vi "KE622x -- Get Trace Buf Elements.vi"(0 "Resource In":refnum<visa-resource-name>, 1 "Check For SCPI Errors? (T)":bool=TRUE, 11 "error in (no error)":errorcluster) -> (4 "Resource Out (dupl)":refnum<visa-resource-name>, 8 "Meas Elements To Return":T1={"Timstamp?"=TRUE, "Reading Num?"=FALSE, "Source Value?"=FALSE, "Compliance?"=TRUE, "Average Voltage?"=FALSE}, 15 "error out":errorcluster)   [LabVIEW 2019, in "Keithley 622x.lvlib"]
uses:
  Keithley 622x.lvlib
  Format/Typedefs/KE622x -- Optional Meas Elements.ctl
panel:
  # "*** NOTE:  \"Average Voltage\"\nis only available for Differential\nConductance measurements."
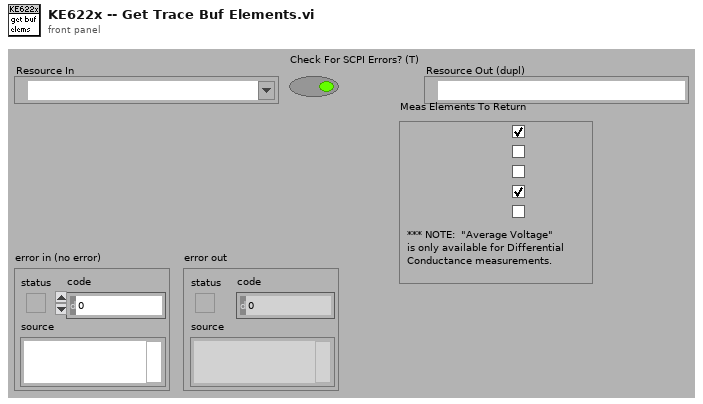
[diagram p1: front panel]
types:
  T1 = typedef "Keithley 622x.lvlib/KE622x -- Optional Meas Elements.ctl" = cluster{"Timstamp?":bool, "Reading Num?":bool, "Source Value?":bool, "Compliance?":bool, "Average Voltage?":bool}
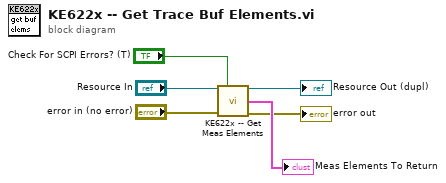
[diagram p0: block diagram]
diagram:
  n1 = call "KE622x -- Get Meas Elements.vi"("Resource In"="Resource In", "Check For SCPI Errors? (T)"="Check For SCPI Errors? (T)", "error in (no error)"="error in (no error)") -> ("Resource Out (dupl)"=→"Resource Out (dupl)":refnum<visa-resource-name>, "Meas Elements To Return"=→"Meas Elements To Return":T1, "error out"=→"error out":errorcluster)  [unwired: 10 in]
